vi "Pre-Build Action - Set Compiler Optimisations.vi"(6 "Top Level/Always Included VIs":path[](array[path]), 7 "Main Destination Path":path, 9 "Target Name":string, 10 "Build Specification Name":string, 11 "Project Path":path) -> (0 "error out":errorcluster)   [LabVIEW 2015, in "Build Tools.lvlib"]
uses:
  Build Tools.lvlib
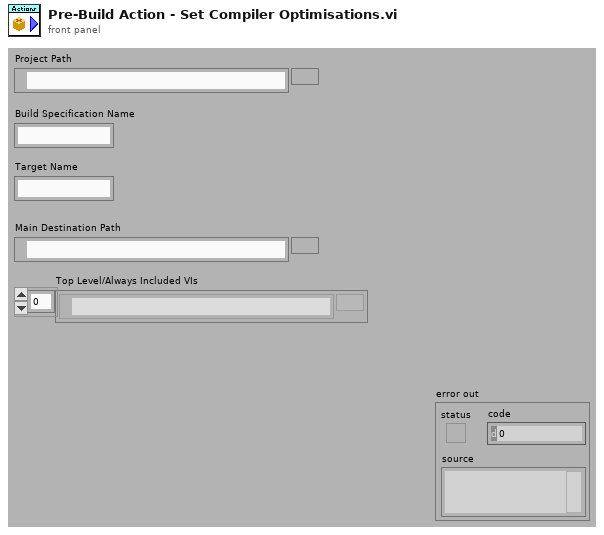
[diagram p1: front panel]
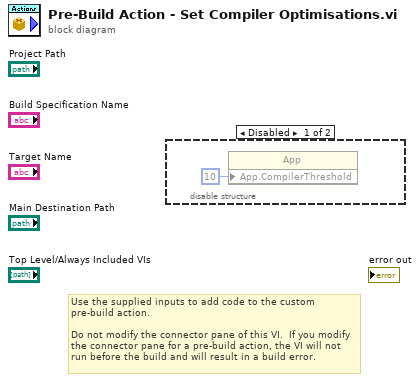
[diagram p0: block diagram]
diagram:
  # "Use the supplied inputs to add code to the custom pre-build action.\n\nDo not modify the connector pane of this VI.  If you modify the connector pane for a pre-build action, the VI will not run before the build and will result in a build error."
  n1 = disable-structure shown="Disabled" {
    frame Disabled {
      n2 = property class="App"("App.CompilerThreshold"=u32 10 ("Application:Compiler Threshold")) -> ()  [unwired: 2 in, 2 out]
    }
    frame Enabled {
    }
  }
